vi "Get_error.vi"(8 "PICam_Error":T1=1 items=["LibraryNotInitialized"=1, "InvalidParameterValue"=2, "UnexpectedNullPointer"=3, "UnexpectedError"=4, "LibraryAlreadyInitialized"=5, "InvalidDemoModel"=6, "CameraAlreadyOpened"=7, "InvalidCameraID"=8, "InvalidHandle"=9, "ParameterValueIsReadOnly"=10, "ParameterHasInvalidValueType"=11, "ParameterDoesNotExist"=12, "ParameterHasInvalidConstraintType"=13, "ParameterValueIsIrrelevant"=14, "DeviceCommunicationFailed"=15, "InvalidEnumeratedType"=16, "EnumerationValueNotDefined"=17, "NotDiscoveringCameras"=18, "AlreadyDiscoveringCameras"=19, "AcquisitionInProgress"=20, "InvalidDemoSerialNumber"=21, "DemoAlreadyConnected"=22, "DeviceDisconnected"=23, "DeviceOpenElsewhere"=24, "ParameterIsNotOnlineable"=25, "ParameterIsNotReadable"=26, "AcquisitionNotInProgress"=27, "InvalidParameterValues"=28, "ParametersNotCommitted"=29, "InvalidAcquisitionBuffer"=30, "InsufficientMemory"=31, "TimeOutOccurred"=32, "AcquisitionUpdatedHandlerRegistered"=33, "NoCamerasAvailable"=34, "InvalidPointer"=35, "InvalidReadoutCount"=36, "InvalidReadoutTimeOut"=37, "InvalidConstraintCategory"=38, "InvalidCount"=39, "DemoNotSupported"=40, "NondestructiveReadoutEnabled"=41, "InvalidOperation"=42, "OperationCanceled"=43, "InvalidAcquisitionState"=44, "NoAccessoriesAvailable"=45, "AccessoryAlreadyOpened"=46, "InvalidAccessoryID"=47, "NotDiscoveringAccessories"=48, "AlreadyDiscoveringAccessories"=49, "ParameterIsNotWaitableStatus"=50, "InvalidWaitableStatusParameterTimeOut"=51, "ShutterOverheated"=52, "CameraFaulted"=53, "CenterWavelengthFaulted"=54], 9 "error in (no error)":errorcluster) -> (1 "error out":errorcluster)   [LabVIEW 2019, in "PICam.lvlib"]
uses:
  PICam.lvlib
  Ctrls/PicamErrors.ctl
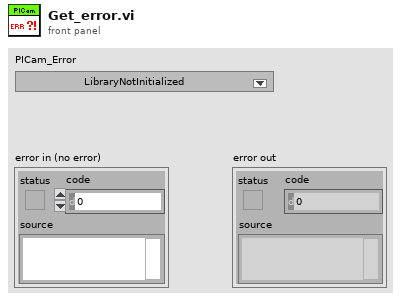
[diagram p1: front panel]
types:
  T1 = typedef "PICam.lvlib/PicamErrors.ctl" = i32
  T2 = typedef "LVStringsAndValuesArrayTypeDef_I32.ctl" = cluster{"String":string, "Value":i32}[]
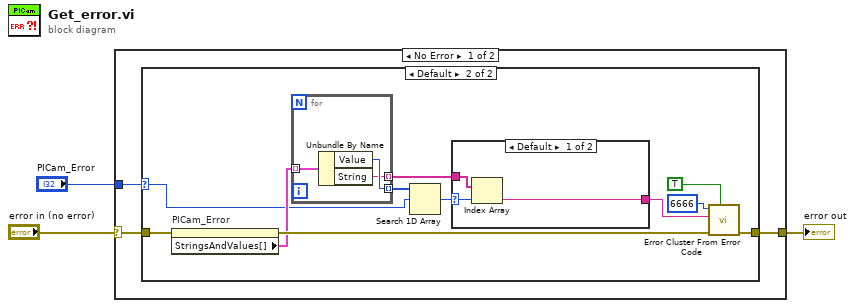
[diagram p0: block diagram]
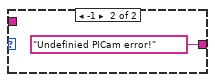
[diagram p3: hidden frame]
diagram:
  n1 = case shown="No Error" "error in (no error)" {
    selector: "error in (no error)" -> [w6 w26]
    tunnel: [w5 w26] -> w2
    tunnel: "PICam_Error" -> [w4 _]
    frame No Error {
      n2 = case shown="Default" w4 {
        selector: w4 -> [_ w9]
        tunnel: w6 -> [w7 w18]
        tunnel: [w7 w14] -> w5
        frame 0 {
          # "no error"
        }
        frame Default {
          n3 = property on="PICam_Error" class="Ring (strict)"(error in=w18) -> (error out=w17:errorcluster, "StringsAndValues[]"=w16:T2)  [unwired: 1 in, 1 out]
          n4 = for {
            tunnel: w16 -> [w25] mode=indexing
            tunnel: [w24] -> w15 mode=indexing
            tunnel: [w23] -> w13 mode=indexing
            n5 = Unbundle By Name(w25) -> ("Value"=w24:i32, "String"=w23:string)
          }
          n6 = Search 1D Array(1D array=w15, element=w9) -> (index of element=w12:i32)  [unwired: 1 in]
          n7 = case shown="Default" w12 {
            selector: w12 -> [w19 _]
            tunnel: w13 -> [w21 _]
            tunnel: [w20 "Undefinied PICam error!"] -> w8
            frame Default {
              n8 = Index Array(array=w21, index=w19) -> (element=w20:string)
            }
            frame -1 {
            }
          }
          n9 = call <vilib>:"Error Cluster From Error Code.vi"("show call chain? (False)"=TRUE, "error in (no error)"=w17, "error message (\"\")"=w8, "error code (0)"=6666) -> ("error out"=w14:errorcluster)  [unwired: 5 in]
        }
      }
    }
    frame Error {
    }
  }
  "error out" <- w2
